vi "Write Control File.vi"(8 "error in (no error)":errorcluster, 10 "Map":map{string, string}(c390), 11 "NIPKG Packager in":refnum<class "NIPKG Packager.lvclass">) -> (0 "error out":errorcluster)   [LabVIEW 2019, in "NIPKG Packager.lvclass"]
uses:
  NIPKG Packager.lvclass
  CLI Output/CLI Output.lvclass
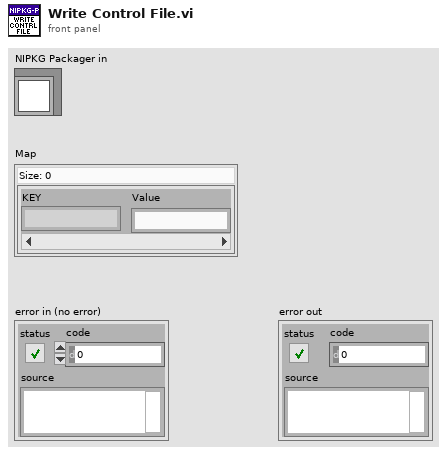
[diagram p1: front panel]
types:
  T1 = enum16{"open", "replace", "create", "open or create", "replace or create", "replace or create with confirmation"}
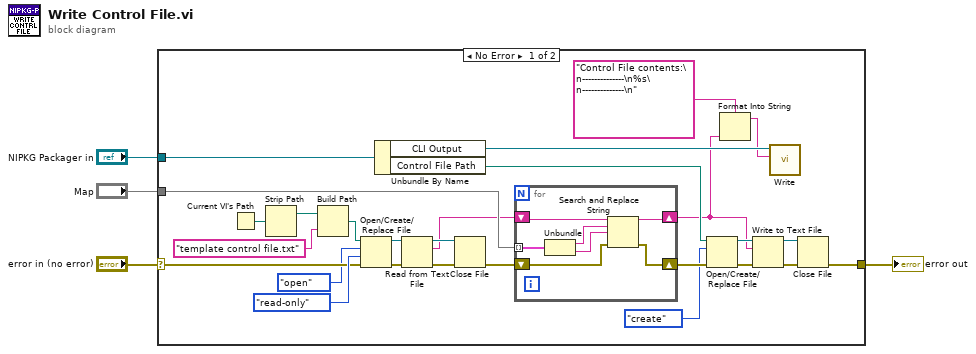
[diagram p0: block diagram]
diagram:
  n1 = case shown="No Error" "error in (no error)" {
    selector: "error in (no error)" -> [w18 w39]
    tunnel: [w27 w39] -> w4
    tunnel: "NIPKG Packager in" -> [w22 _]
    tunnel: "Map" -> [w31 _]
    frame No Error {
      n2 = Current VI's Path() -> (path=w13:path)
      n3 = Strip Path(path=w13) -> (stripped path=w12:path)  [unwired: 1 out]
      n4 = Build Path(base path=w12, name or relative path="template control file.txt") -> (appended path=w11:path)
      n5 = Open/Create/Replace File(file path (use dialog)=w11, error in=w18, operation (0:open)=T1."open", access (0:read/write)=enum16{"read/write", "read-only", "write-only"}."read-only") -> (refnum out=w20:refnum<file>, error out=w16:errorcluster)  [unwired: 2 in, 1 out]
      n6 = Unbundle By Name(w22) -> ("CLI Output"=w8:refnum<class "CLI Output.lvclass">, "Control File Path"=w9:path)
      n7 = Read from Text File(file (use dialog)=w20, error in=w16) -> (refnum out=w25:refnum<file>, text=w15:string, error out=w19:errorcluster)  [unwired: 2 in, 1 out]
      n8 = Close File(refnum=w25, error in=w19) -> (error out=w14:errorcluster)  [unwired: 1 out]
      n9 = for {
        shift-right: [w36] -> w7
        shift-left: w15 -> [w37]
        tunnel: w31 -> [w38] mode=indexing
        shift-right: [w35] -> w30
        shift-left: w14 -> [w34]
        n10 = Unbundle(w38) -> ("KEY"=w33:string, "Value"=w32:string)
        n11 = Search and Replace String(input string=w37, search string=w33, replace string=w32, error in=w34) -> (result string=w36:string, error out=w35:errorcluster)  [unwired: 4 in, 2 out]
      }
      n12 = Open/Create/Replace File(file path (use dialog)=w9, error in=w30, operation (0:open)=T1."create") -> (refnum out=w28:refnum<file>, error out=w21:errorcluster)  [unwired: 3 in, 1 out]
      n13 = Format Into String(format string="Control File contents:\n--------------\n%s\n--------------\n", w7) -> (resulting string=w6:string)  [unwired: 2 in, 1 out]
      n14 = Write to Text File(file (use dialog)=w28, text=w7, error in=w21) -> (refnum out=w29:refnum<file>, error out=w26:errorcluster)  [unwired: 1 in, 1 out]
      n15 = call-dynamic "Write.vi"("String"=w6, "CLI Output in"=w8) -> ()  [unwired: 8 in, 2 out]
      n16 = Close File(refnum=w29, error in=w26) -> (error out=w27:errorcluster)  [unwired: 1 out]
    }
    frame Error {
    }
  }
  "error out" <- w4
